vi "Test ZXing QR Code Detector.vi"(11 "Test Case In":refnum<class "02_FeatureDetection.lvclass">) -> (0 "error out":errorcluster, 3 "Test Case Out":refnum<class "02_FeatureDetection.lvclass">)   [LabVIEW 2020, in "test.lvlib" / "02_FeatureDetection.lvclass"]
uses:
  02_FeatureDetection.lvclass
  C:/Program Files (x86)/National Instruments/LabVIEW 2020/vi.lib/Astemes/LUnit/Test Case.lvclass
  <vilib>/picture/picture.llb/imagedata.ctl
  common/Quad Corners.ctl
  common/Image Point (Float).ctl
  feature_detection/ZXing/ZXing.lvclass/ZXing.ctl
  <vilib>/Astemes/LUnit/Test Case.lvclass/Test Case.ctl
  image/New Image (ARGB Preallocated).vi
  image/Copy Pixmap to Image (ARGB Flatten Mask).vi
  feature_detection/ZXing/Read Barcodes (ARGB).vi
  c620ff27-3bdc-43ee-ae28-79191c7efa9c.vi
  image/New Image (Greyscale Preallocated).vi
  image/Copy Pixmap to Image (Greyscale Flatten Mask).vi
  feature_detection/ZXing/Read Barcodes (Greyscale).vi
  81cff08c-ad27-40c1-b34f-f5a0f1f6849e.vi
  image/New Image (ARGB Preallocated).vi/3321fa97-f432-4e1e-8db9-a0df79aed21b.vi
  image/ARGB Colour to U32 Pixel Value.vi
  image/Copy Pixmap to Image (ARGB Flatten Mask).vi/7d03ccf7-b889-4e8d-9f2a-57831e73dbde.vi
  feature_detection/ZXing/Read Barcodes (ARGB).vi/a90e4b0e-e65a-4d68-81f3-9c053758d966.vi
  <vilib>/Astemes/LUnit/Core/LUnit Test Case/Private/Append Pass Result.vi
  <vilib>/Astemes/LUnit/Core/LUnit Test Case/Private/Append Fail Result.vi
  c620ff27-3bdc-43ee-ae28-79191c7efa9c.vi/9c5d11cd-9439-4240-a1ee-d9baace9c924.vi
  image/New Image (Greyscale Preallocated).vi/6598b9e0-8a08-46f5-91fd-ca1b87217137.vi
  image/Copy Pixmap to Image (Greyscale Flatten Mask).vi/f0818824-bd55-4656-87f2-fcc208e7cf24.vi
  feature_detection/ZXing/Read Barcodes (Greyscale).vi/a90e4b0e-e65a-4d68-81f3-9c053758d966.vi
  81cff08c-ad27-40c1-b34f-f5a0f1f6849e.vi/9c5d11cd-9439-4240-a1ee-d9baace9c924.vi
  image/FixPixmap.vi
  common/Break on NILRT-ARM32.vi
  <vilib>/Astemes/LUnit/Core/LUnit Test Case/Private/Run In UI.vi
  image/Default8bitColourMap.vi
  <vilib>/Utility/error.llb/Clear Errors.vi
  <vilib>/Utility/error.llb/Error Cluster From Error Code.vi
  feature_detection/ZXing/ZXing.lvclass
  image/image.lvlib
  common/common.lvlib
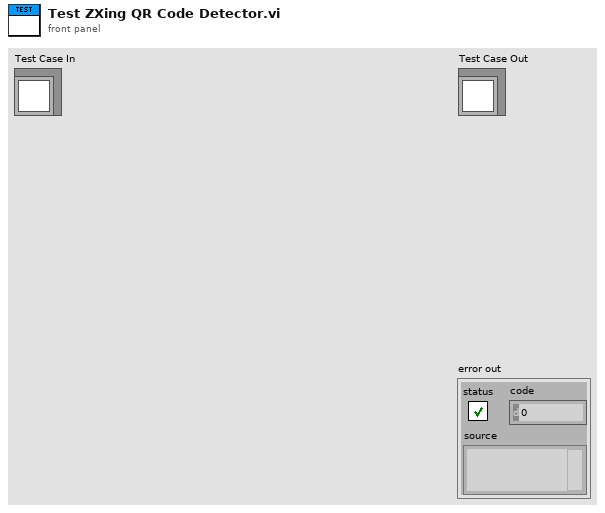
[diagram p1: front panel]
types:
  T1 = typedef "common.lvlib/Quad Corners.ctl" = cluster{"Bottom Left":T2, "Bottom Right":T2, "Top Right":T2, "Top Left":T2}
  T2 = typedef "common.lvlib/Image Point (Float).ctl" = cluster{"x":dbl, "y":dbl}
  T3 = typedef "imagedata.ctl" = cluster{"image type":i32, "image depth":i32, "image":u8[], "mask":u8[], "colors":u32[], "Rectangle":cluster{"left":i16, "top":i16, "right":i16, "bottom":i16}}
  T4 = typedef "image.lvlib/ARGB Image.ctl" = refnum<data-value>
  T5 = typedef "feature_detection.lvlib/ZXing.lvclass/Barcode.ctl" = cluster{"Is Valid":bool, "Text":string, "Format":T6, "Content Type":T7, "Corners":T1, "Orientation":i32, "Bytes":u8[], "Bytes ECI":u8[], "Symbol Identifier":string, "Has ECI":bool, "Is Mirrored":bool, "Is Inverted":bool, "Is Part of Sequence":bool, "EC Level":string, "Version":string, "Error Message":string, "Error Type":T8, "Line Count":i32, "Sequence Size":i32, "Sequence Index":i32, "Sequence ID":string, "Country":string, "Add On":string, "Price":string, "Issue Number":string}
  T6 = typedef "feature_detection.lvlib/ZXing.lvclass/Format.ctl" = enum8{"Aztec", "Codabar", "Code 39", "Code 93", "Code 128", "Data Bar", "Data Bar Expanded", "Data Matrix", "EAN 8", "EAN 13", "ITF", "Maxi Code", "PDF417", "QR Code", "UPCA", "UPCE", "Micro QR Code", "RM QR Code", "DX Film Edge", "Data Bar Limited"}
  T7 = typedef "feature_detection.lvlib/ZXing.lvclass/Content Type.ctl" = enum8{"Text", "Binary", "Mixed", "GS1", "ISO15434", "UnknownECI"}
  T8 = typedef "feature_detection.lvlib/ZXing.lvclass/Error Type.ctl" = u8
  T9 = typedef "image.lvlib/Greyscale Image.ctl" = refnum<data-value>
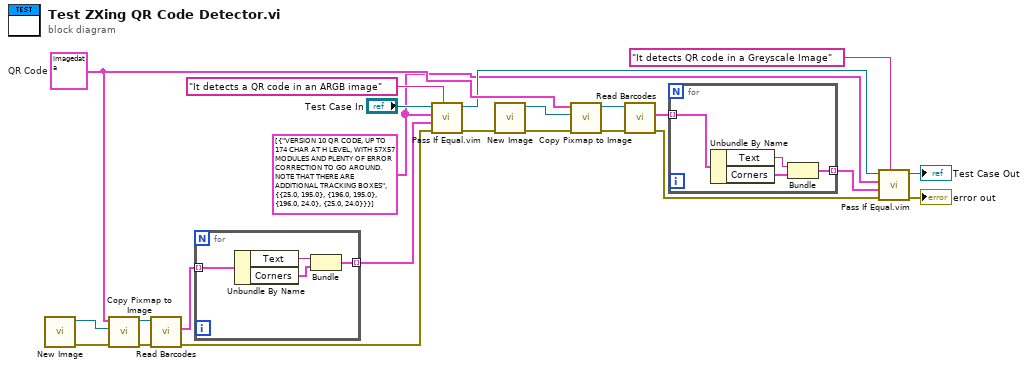
[diagram p0: block diagram]
diagram:
  w1 = cluster{"Text":string, "Corners":T1}[] [{"Text"="VERSION 10 QR CODE, UP TO 174 CHAR AT H LEVEL, WITH 57X57 MODULES AND PLENTY OF ERROR CORRECTION TO GO AROUND.  NOTE THAT THERE ARE ADDITIONAL TRACKING BOXES", "Corners"={"Bottom Left"={"x"=25.0, "y"=195.0}, "Bottom Right"={"x"=196.0, "y"=195.0}, "Top Right"={"x"=196.0, "y"=24.0}, "Top Left"={"x"=25.0, "y"=24.0}}}] ("Array")
  w18 = T3 {"image type"=0, "image depth"=24, "image"=array[145200 elements], "mask"=[], "colors"=[], "Rectangle"={"left"=0, "top"=0, "right"=220, "bottom"=220}}  # QR Code
  n1 = call-poly "New Image.vi"() -> ("error out"=w21:errorcluster, "ARGB Image"=w22:T4)  [unwired: 10 in]
  n2 = call-poly "Copy Pixmap to Image.vi"("error in (no error)"=w21, "ARGB Image Destination in"=w22, "Pixmap Image Data"=w18) -> ("error out"=w20:errorcluster, "ARGB Image Destination"=w3:T4)  [unwired: 7 in]
  n3 = call-poly "Read Barcodes.vi"("error in (no error)"=w20, "ARGB Image in"=w3) -> ("error out"=w2:errorcluster, "Barcodes"=w7:T5[])  [unwired: 7 in, 1 out]
  n4 = for {
    tunnel: w7 -> [w27] mode=indexing
    tunnel: [w25] -> w4 mode=indexing
    n5 = Unbundle By Name(w27) -> ("Text"=w26:string, "Corners"=w24:T1)
    n6 = Bundle("Text"=w26, "Corners"=w24) -> (w25:cluster{"Text":string, "Corners":T1})  [unwired: 1 in]
  }
  n7 = call "Pass If Equal.vim"("Description"="It detects a QR code in an ARGB image", "error in (no error)"=w2, "Actual"=w4, "Expected"=w1, "LUnit Test Case In"="Test Case In") -> ("error out"=w13:errorcluster, "LUnit Test Case Out"=w12:refnum<class "02_FeatureDetection.lvclass">)  [unwired: 5 in]
  n8 = call-poly "New Image.vi"("error in (no error)"=w13) -> ("error out"=w17:errorcluster, "Greyscale Image"=w16:T9)  [unwired: 9 in]
  n9 = call-poly "Copy Pixmap to Image.vi"("error in (no error)"=w17, "Greyscale Image Destination in"=w16, "Pixmap Image Data"=w18) -> ("error out"=w14:errorcluster, "Greyscale Image Destination"=w15:T9)  [unwired: 7 in]
  n10 = call-poly "Read Barcodes.vi"("error in (no error)"=w14, "Greyscale Image in"=w15) -> ("error out"=w10:errorcluster, "Barcodes"=w6:T5[])  [unwired: 7 in, 1 out]
  n11 = for {
    tunnel: w6 -> [w31] mode=indexing
    tunnel: [w28] -> w5 mode=indexing
    n12 = Unbundle By Name(w31) -> ("Text"=w30:string, "Corners"=w29:T1)
    n13 = Bundle("Text"=w30, "Corners"=w29) -> (w28:cluster{"Text":string, "Corners":T1})  [unwired: 1 in]
  }
  n14 = call "Pass If Equal.vim"("Description"="It detects QR code in a Greyscale Image", "error in (no error)"=w10, "Actual"=w5, "Expected"=w1, "LUnit Test Case In"=w12) -> ("error out"=→"error out":errorcluster, "LUnit Test Case Out"=→"Test Case Out":refnum<class "02_FeatureDetection.lvclass">)  [unwired: 5 in]
